vi "主模块.vi"() -> ()   [LabVIEW 2017]
panel:
  in  "simulink":bool
  in  "模态、幅响应分析":bool
  in  "阻抗分析":bool
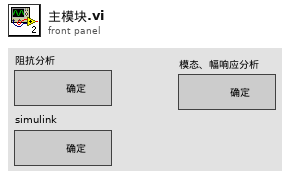
[diagram p1: front panel]
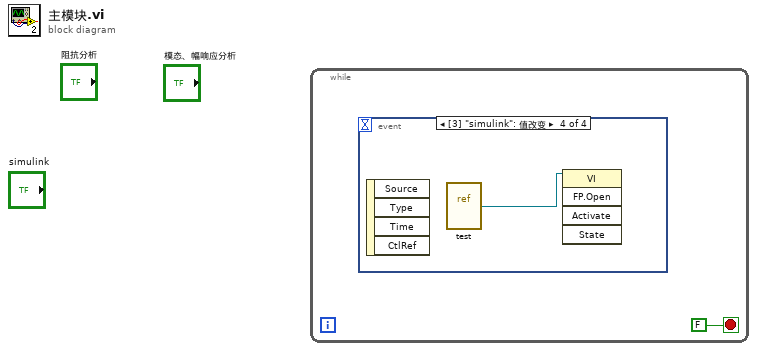
[diagram p0: block diagram]
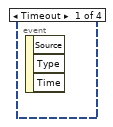
[diagram p2: hidden frame]
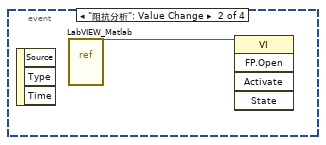
[diagram p3: hidden frame]
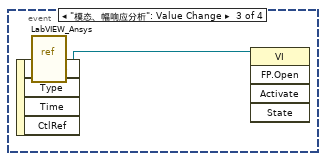
[diagram p4: hidden frame]
diagram:
  n1 = while {
    stop <- FALSE stop-if-true
    n2 = event shown="[3] \"simulink\": 值改变" {
      selector: _ -> [_ _ _ _]
      dyn-events: _ -> [_ _ _ _]
      timeout: _ -> [_ _ _ _]
      event Timeout {
        n3 = event-data() -> ()  [unwired: 1 in, 3 out]
      }
      event "阻抗分析": Value Change {
        n4 = event-data() -> ()  [unwired: 1 in, 3 out]
        n5 = vi-ref "LabVIEW_Matlab.vi"() -> (w2:refnum<vi>)
        n6 = invoke class="VI" method="FP.Open"(reference=w2) -> ()  [unwired: 4 in, 5 out]
      }
      event "模态、幅响应分析": Value Change {
        n7 = event-data() -> ()  [unwired: 1 in, 4 out]
        n8 = vi-ref "LabVIEW_Ansys.vi"() -> (w3:refnum<vi>)
        n9 = invoke class="VI" method="FP.Open"(reference=w3) -> ()  [unwired: 4 in, 5 out]
      }
      event "simulink": Value Change {
        n10 = event-data() -> ()  [unwired: 1 in, 4 out]
        n11 = vi-ref "test.vi"() -> (w4:refnum<vi>)
        n12 = invoke class="VI" method="FP.Open"(reference=w4) -> ()  [unwired: 4 in, 5 out]
      }
    }
  }
